vi "Load Settings from XML.vi"(8 "error in (no error)":T5 caption="entrée d'erreur (pas d'erreur)", 11 "Paramètres en entrée":T1) -> (0 "error out":T5 caption="sortie d'erreur", 3 "Paramètres en sortie":T1)   [LabVIEW 2020, in "Settings.lvlib"]
doc: "Tente de charger d'anciens paramètres utilisateur à partir d'un fichier XML.\n\nCe VI ne génèrera pas d'erreur. Si aucun fichier XML ne peut être chargé et analysé, le VI renverra les paramètres par défaut."
uses:
  Settings.lvlib
  Settings.ctl
  Acquisition/Hardware Configuration.ctl
  Acquisition/Signal Type.ctl
  Logging/Logging Configuration.ctl
  <vilib>/Utility/xml.llb/Read From XML File(string).vi
  <vilib>/Utility/xml.llb/Write to XML File(string).vi
  Acquisition/Acquisition.lvlib
  Logging/Logging.lvlib
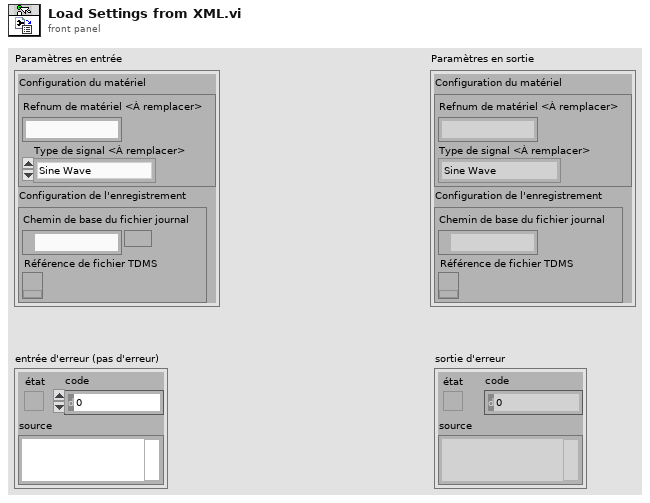
[diagram p1: front panel]
types:
  T1 = typedef "Settings.lvlib/Settings.ctl" = cluster{"Configuration du matériel":T2, "Configuration de l'enregistrement":T4}
  T2 = typedef "Acquisition.lvlib/Hardware Configuration.ctl" = cluster{"Refnum de matériel <À remplacer>":string, "Type de signal <À remplacer>":T3}
  T3 = typedef "Acquisition.lvlib/Signal Type.ctl" = enum16{"Sine Wave", "Square with Noise", "Signal triangulaire", "Simulation DAQ"}
  T4 = typedef "Logging.lvlib/Logging Configuration.ctl" = cluster{"Chemin de base du fichier journal":path, "Référence de fichier TDMS":refnum<k34>}
  T5 = cluster{"état":bool, "code":i32, "source":string}
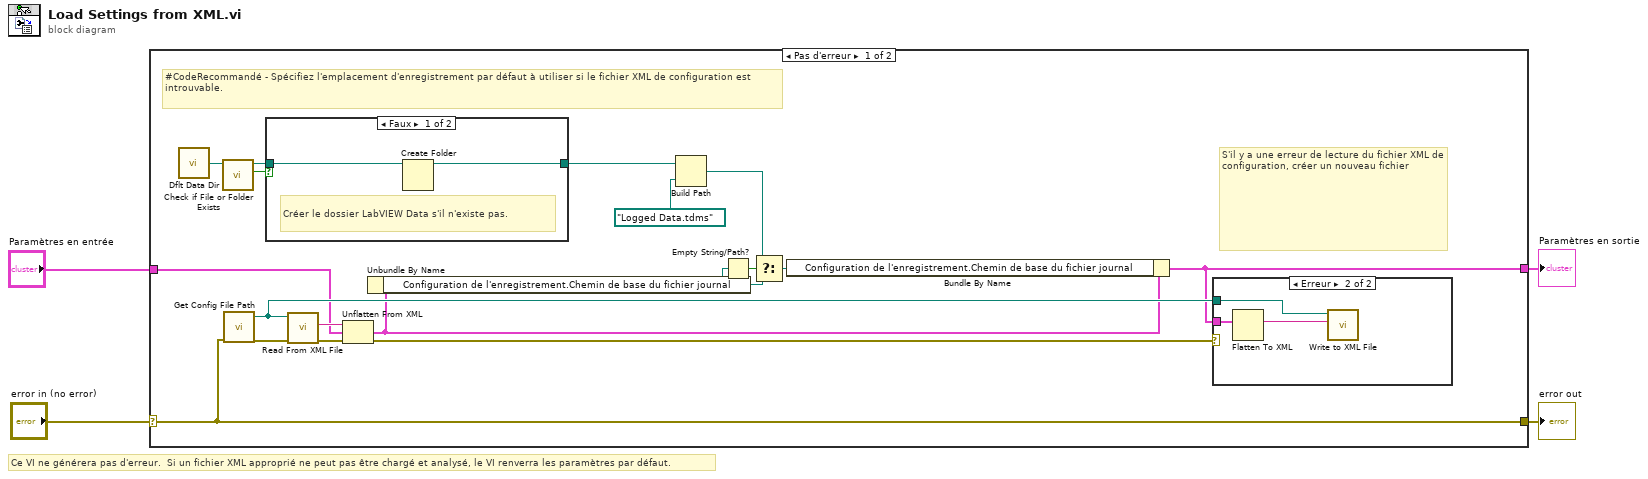
[diagram p0: block diagram]
diagram:
  # "Ce VI ne générera pas d'erreur.  Si un fichier XML approprié ne peut pas être chargé et analysé, le VI renverra les paramètres par défaut."
  n1 = case shown="Pas d'erreur" "error in (no error)" {
    selector: "error in (no error)" -> [w20 w30]
    tunnel: [w20 w30] -> w3
    tunnel: "Paramètres en entrée" -> [w15 w29]
    tunnel: [w9 w29] -> w1
    frame No Error {
      # "S'il y a une erreur de lecture du fichier XML de configuration, créer un nouveau fichier"
      # "#CodeRecommandé - Spécifiez l'emplacement d'enregistrement par défaut à utiliser si le fichier XML de configuration est introuvable."
      n2 = call <vilib>:"Dflt Data Dir.vi"() -> ("App:Default Data Directory"=w8:path)
      n3 = call <vilib>:"Check if File or Folder Exists.vi"("path"=w8) -> ("file or folder exists?"=w7:bool, "dup path"=w6:path)  [unwired: 8 in, 1 out]
      n4 = call "Get Config File Path.vi"("error in (no error)"=w20) -> ("error out"=w22:T5, "Chemin du fichier XML"=w18:path)  [unwired: 9 in]
      n5 = case shown="Faux" w7 {
        tunnel: w6 -> [w24 w25]
        tunnel: [w23 w25] -> w5
        frame False {
          # "Créer le dossier LabVIEW Data s'il n'existe pas."
          n6 = Create Folder(path (use dialog)=w24) -> (created path=w23:path)  [unwired: 2 in, 2 out]
        }
        frame True {
        }
      }
      n7 = call-poly <vilib>:"Read From XML File.vi"("error in (no error)"=w22, "XML File Path"=w18) -> ("error out"=w17:errorcluster, "XML Elements"=w21:string)  [unwired: 7 in, 1 out]
      n8 = Unflatten From XML(xml string=w21, type=w15, error in (no error)=w17) -> (value=w11:T1, error out=w16:errorcluster)
      n9 = Unbundle By Name(w11) -> ("Configuration de l'enregistrement.Chemin de base du fichier journal"=w13:path)
      n10 = Build Path(base path=w5, name or relative path=path "Logged Data.tdms" ("App:Default Data Directory")) -> (appended path=w12:path)
      n11 = Empty String/Path?(string/path=w13) -> (empty?=w14:bool)
      n12 = Select(t=w12, s=w14, f=w13) -> (s? t:f=w10:path)
      n13 = Bundle By Name(cluster=w11, "Configuration de l'enregistrement.Chemin de base du fichier journal"=w10) -> (w9:T1)
      n14 = case shown="Erreur" w16 {
        tunnel: w9 -> [_ w28]
        tunnel: w18 -> [_ w26]
        frame No Error {
        }
        frame Error {
          n15 = Flatten To XML(6:w28) -> (2:w27:string)
          n16 = call-poly <vilib>:"Write to XML File.vi"("XML Input"=w27, "XML File Path"=w26) -> ()  [unwired: 7 in, 3 out]
        }
      }
    }
    frame Error {
    }
  }
  "error out" <- w3
  "Paramètres en sortie" <- w1
